vi "Bead tester-reload avi.vi"() -> ()   [LabVIEW 2020]
uses:
  <vilib>/vision/Avi.llb/IMAQ AVI2 Codec Path.ctl
  <vilib>/vision/NI_Vision_Development_Module.lvlib
panel:
  out "Numeric":i32
  out "Image 2":T1(plugin-control)
  out "Number of Frames":u32
  out "Image":T1(plugin-control)
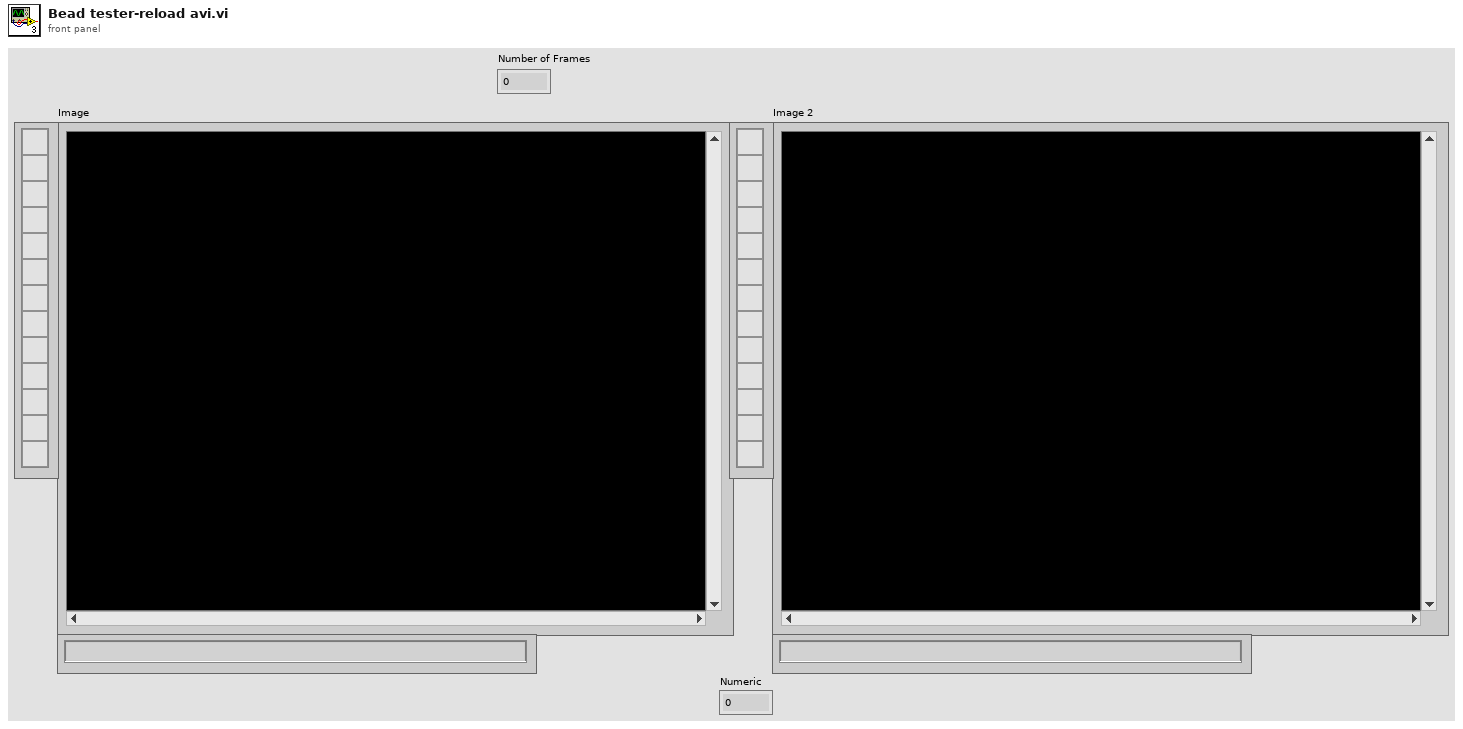
[diagram p1: front panel]
types:
  T1 = typedef "IMAQ Image.ctl" = refnum<image>
  T2 = typedef "Image Type" = u32
  T3 = typedef "IMAQ AVI2 Codec Path.ctl" = u32
  T4 = typedef "IMAQ AVI2 Refnum.ctl" = refnum<k20>
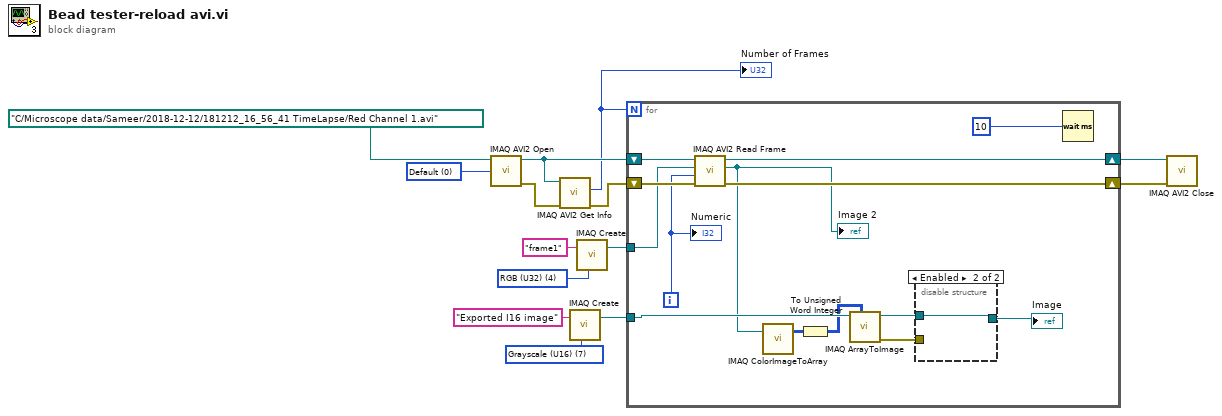
[diagram p0: block diagram]
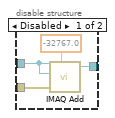
[diagram p2: hidden frame]
diagram:
  w3 = T2 7 items=["Grayscale (U8)", "Grayscale (I16)", "Grayscale (SGL)", "Complex (CSG)", "RGB (U32)", "HSL (U32)", "RGB (U64)", "Grayscale (U16)"] ("Image Type")
  w4 = T3 0 items=["Default", "System", "Built in Vision"] ("Codec Source")
  w8 = T2 4 items=["Grayscale (U8)", "Grayscale (I16)", "Grayscale (SGL)", "Complex (CSG)", "RGB (U32)", "HSL (U32)", "RGB (U64)", "Grayscale (U16)"] ("Image Type")
  n1 = call "IMAQ AVI2 Open"("Codec Source"=w4, "AVI File Path"=path "C:/Microscope data/Sameer/2018-12-12/181212_16_56_41 TimeLapse/Red Channel 1.avi" ("AVI Path")) -> ("error out"=w10:errorcluster, "AVI Refnum"=w11:T4)  [unwired: 8 in]
  n2 = call "IMAQ AVI2 Get Info"("error in (no error)"=w10, "AVI Refnum"=w11) -> ("error out"=w9:errorcluster, "Number of Frames"=w5:u32)  [unwired: 5 in, 3 out]
  "Number of Frames" <- w5
  n3 = call "IMAQ Create"("Image Name"="Exported I16 image", "Image Type"=w3) -> ("New Image"=w1:T1)  [unwired: 2 in, 2 out]
  n4 = call "IMAQ Create"("Image Name"="frame1", "Image Type"=w8) -> ("New Image"=w6:T1)  [unwired: 3 in, 1 out]
  n5 = for {
    N: w5 -> [_]
    tunnel: w6 -> [w24]
    shift-right: [w28] -> w13
    shift-left: w11 -> [w26]
    shift-right: [w27] -> w12
    shift-left: w9 -> [w25]
    tunnel: w1 -> [w17]
    i -> [w23]
    n6 = call "IMAQ AVI2 Read Frame"("error in (no error)"=w25, "Frame Number"=w23, "Image"=w24, "AVI Refnum"=w26) -> ("error out"=w27:errorcluster, "Image Out"=w16:T1, "AVI Refnum (duplicate)"=w28:T4)  [unwired: 5 in]
    "Image 2" <- w16
    n7 = call "IMAQ ColorImageToArray"("Image"=w16) -> ("Image Pixels (U32)"=w19:u32[][])  [unwired: 2 in, 3 out]
    n8 = To Unsigned Word Integer(number=w19) -> (unsigned 16bit integer=w15:u16[][])
    n9 = call "IMAQ ArrayToImage"("Image Pixels (U16)"=w15, "Image"=w17) -> ("error out"=w20:errorcluster, "Image Out"=w21:T1)  [unwired: 8 in]
    n10 = disable-structure shown="Enabled" {
      disable-tunnel: w21 -> [w32 w33]
      disable-tunnel: w20 -> [w31 _]
      disable-tunnel: [w29 w33] -> w18
      frame Disabled {
        n11 = call "IMAQ Add"("Image Src A"=w32, "Constant"=-32767.0, "Image Dst"=w32, "error in (no error)"=w31) -> ("Image Dst Out"=w29:T1)  [unwired: 3 in, 1 out]
      }
      frame Enabled {
      }
    }
    "Image" <- w18
    n12 = Wait (ms)(milliseconds to wait=u32 10) -> ()  [unwired: 1 out]
    "Numeric" <- w23
  }
  n13 = call "IMAQ AVI2 Close"("error in (no error)"=w12, "AVI Refnum"=w13) -> ()  [unwired: 9 in, 1 out]
